vi "Duplicate_AO_WF.vi"(8 "error in (no error)":errorcluster) -> (0 "error out":errorcluster)   [LabVIEW 2025]
uses:
  <vilib>/Waveform/WDTOps.llb/WDT Append Waveforms DBL.vi
panel:
  out "AO WF":waveform(dbl)[](graph) caption="Output Waveform"
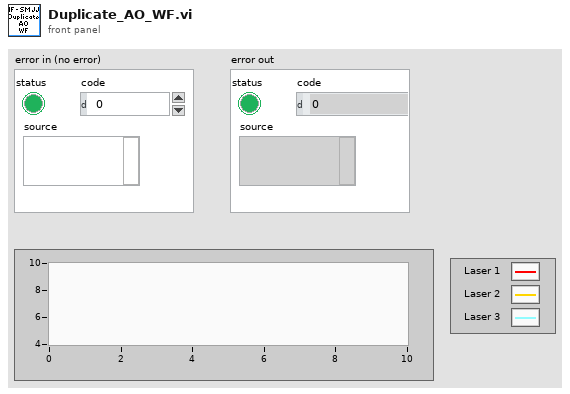
[diagram p1: front panel]
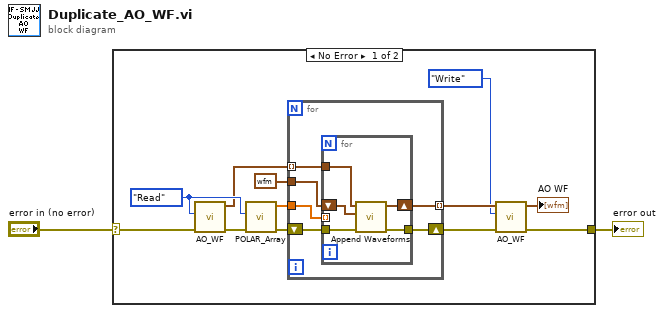
[diagram p0: block diagram]
diagram:
  n1 = case shown="No Error" "error in (no error)" {
    selector: "error in (no error)" -> [w9 w26]
    tunnel: [w4 w26] -> w2
    frame No Error {
      w12 = enum16{"Write", "Read"}."Read" ("Action")
      n2 = call "AO_WF.vi"("error in"=w9, "Action"=w12) -> ("error out"=w10:errorcluster, "AO WF"=w11:waveform(dbl)[])  [unwired: 8 in]
      n3 = call "POLAR_Array.vi"("error in"=w10, "Action"=w12) -> ("error out"=w14:errorcluster, "Pockels_Array"=w13:dbl[])  [unwired: 8 in]
      n4 = for {
        tunnel: w13 -> [w19]
        tunnel: w11 -> [w18] mode=indexing
        tunnel: [w17] -> w8 mode=indexing
        tunnel: waveform(i32) {"t0"=timestamp(0 s since 1904-01-01), "dt"=1.0, "Y"=[]} ("waveform out") -> [w15]
        shift-right: [w16] -> w5
        shift-left: w14 -> [w20]
        n5 = for {
          tunnel: w18 -> [w23]
          shift-right: [w25] -> w17
          shift-left: w15 -> [w24]
          tunnel: w20 -> [w22]
          tunnel: [w21] -> w16
          tunnel: w19 -> [_] mode=indexing
          n6 = call-poly <vilib>:"Append Waveforms.vi"("error in (no error)"=w22, "waveform B"=w24, "waveform A"=w23) -> ("error out"=w21:errorcluster, "waveform out"=w25:waveform(dbl))  [unwired: 7 in]
        }
      }
      n7 = call "AO_WF.vi"("error in"=w5, "Action"=enum16{"Write", "Read"}."Write", "AO WF"=w8) -> ("error out"=w4:errorcluster, "AO WF"=→"AO WF":waveform(dbl)[])  [unwired: 7 in]
    }
    frame Error {
    }
  }
  "error out" <- w2
